vi "SwitchChart.vi"(8 "error in (no error)":errorcluster, 10 "Switch":bool, 11 "Linear_Task in":refnum<class "Linear_Task.lvclass">) -> (0 "error out":errorcluster, 3 "Linear_Task out":refnum<class "Linear_Task.lvclass">)   [LabVIEW 2025, in "Linear_Task.lvlib" / "Linear_Task.lvclass"]
uses:
  Linear_Task.lvclass
  Linear_Task.lvclass/Linear_Task.ctl
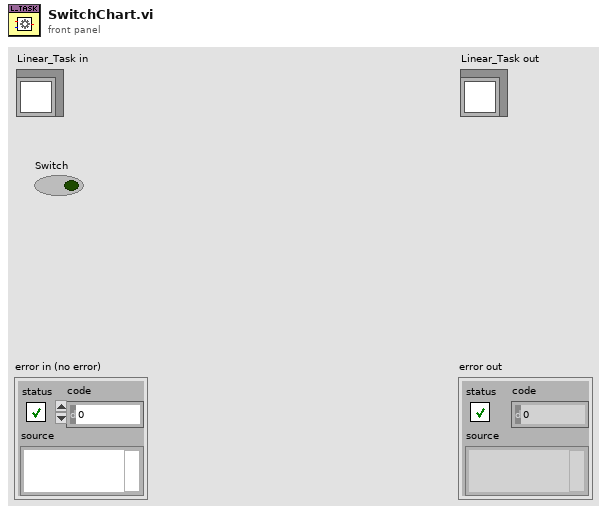
[diagram p1: front panel]
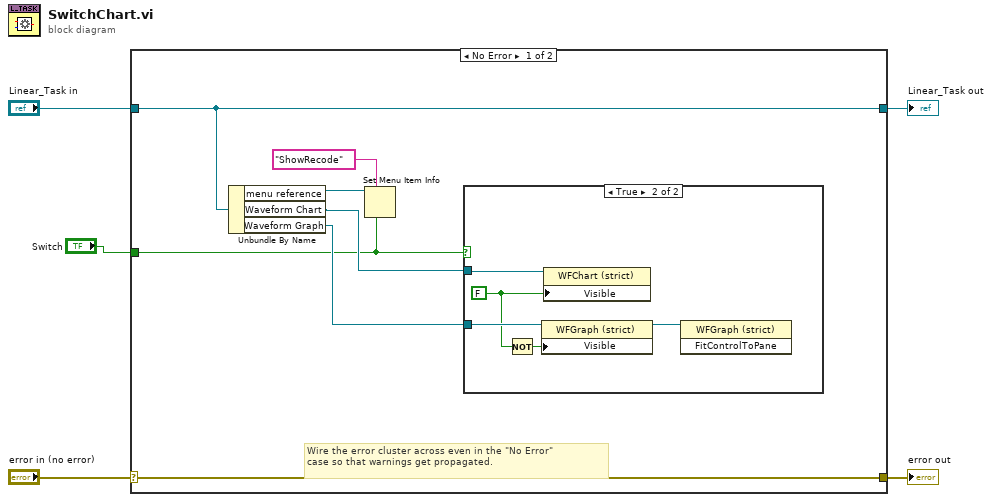
[diagram p0: block diagram]
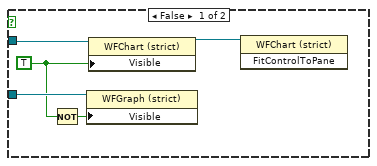
[diagram p2: hidden frame]
diagram:
  n1 = case shown="No Error" "error in (no error)" {
    selector: "error in (no error)" -> [w12 w24]
    tunnel: [w12 w24] -> w4
    tunnel: [w7 w23] -> w2
    tunnel: "Linear_Task in" -> [w7 w23]
    tunnel: "Switch" -> [w6 _]
    frame No Error {
      # "Wire the error cluster across even in the \"No Error\"\ncase so that warnings get propagated."
      n2 = Unbundle By Name(w7) -> ("menu reference"=w11:refnum<k9>, "Waveform Chart"=w9:refnum<vi>, "Waveform Graph"=w8:refnum<vi>)
      n3 = Set Menu Item Info(6:w6, 7:"ShowRecode" ("item tag"), 11:w11) -> ()  [unwired: 4 in, 2 out]
      n4 = case shown="True" w6 {
        tunnel: w9 -> [w17 w22]
        tunnel: w8 -> [w16 w21]
        frame False {
          w15 = TRUE ("Visible")
          n5 = Not(x=w15) -> (.not. x?=w14:bool)
          n6 = property class="WFGraph (strict)"(reference=w16, "Visible"=w14) -> ()  [unwired: 1 in, 2 out]
          n7 = property class="WFChart (strict)"(reference=w17, "Visible"=w15) -> (reference out=w13:refnum<vi>)  [unwired: 1 in, 1 out]
          n8 = invoke class="WFChart (strict)" method="FitControlToPane"(reference=w13) -> ()  [unwired: 2 in, 3 out]
        }
        frame True {
          w20 = FALSE ("Visible")
          n9 = Not(x=w20) -> (.not. x?=w19:bool)
          n10 = property class="WFGraph (strict)"(reference=w21, "Visible"=w19) -> (reference out=w18:refnum<vi>)  [unwired: 1 in, 1 out]
          n11 = property class="WFChart (strict)"(reference=w22, "Visible"=w20) -> ()  [unwired: 1 in, 2 out]
          n12 = invoke class="WFGraph (strict)" method="FitControlToPane"(reference=w18) -> ()  [unwired: 2 in, 3 out]
        }
      }
    }
    frame Error {
    }
  }
  "error out" <- w4
  "Linear_Task out" <- w2
